vi "SpinAuxsAuto.vi"(6 "IntakeSpd":dbl, 7 "Time":dbl, 8 "error in":errorcluster, 9 "FeedSpd":dbl, 10 "Beltspd":dbl, 11 "ShootSpd":dbl) -> (0 "error out":errorcluster, 3 "Done":bool)   [LabVIEW 2020]
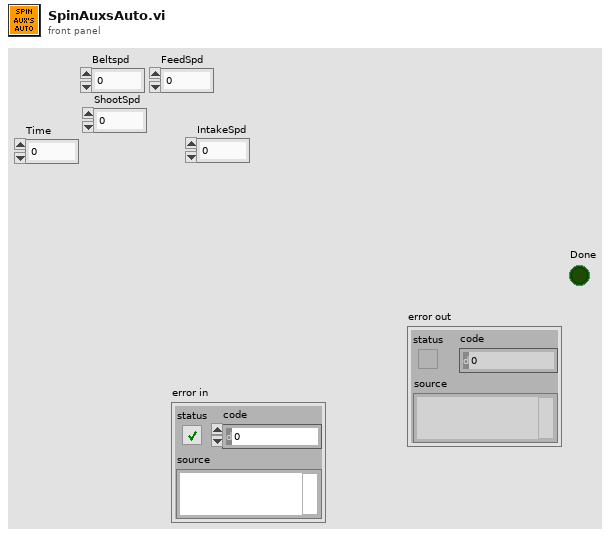
[diagram p1: front panel]
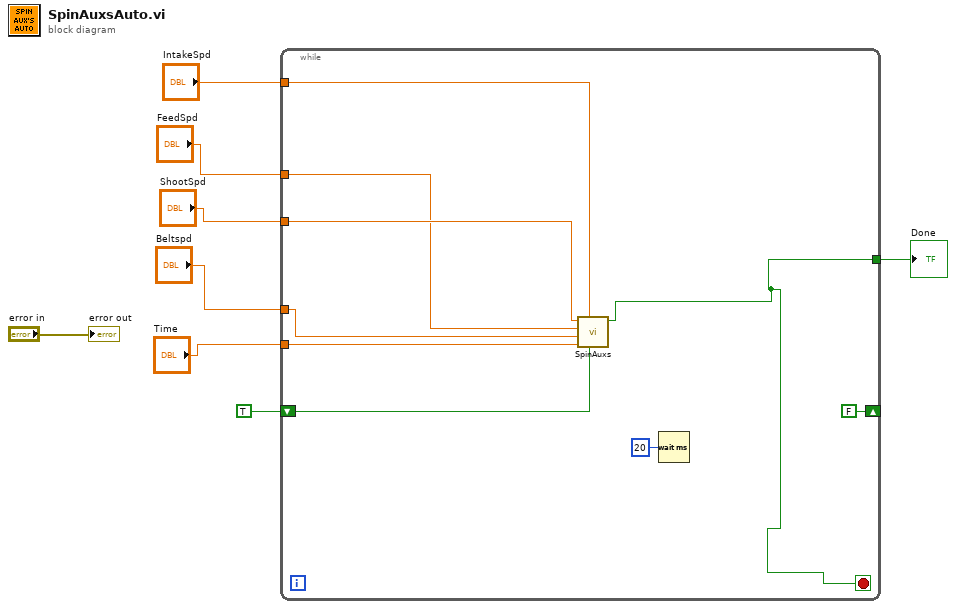
[diagram p0: block diagram]
diagram:
  n1 = while {
    tunnel: [w10] -> w7
    tunnel: "Beltspd" -> [w12]
    tunnel: "ShootSpd" -> [w14]
    tunnel: "FeedSpd" -> [w13]
    shift-right: [FALSE] -> _
    shift-left: TRUE -> [w11]
    tunnel: "Time" -> [w15]
    tunnel: "IntakeSpd" -> [w9]
    stop <- w10 stop-if-true
    n2 = call "SpinAuxs.vi"("Init"=w11, "IntakeSpeed"=w9, "Time"=w15, "BeltSpeed"=w12, "FeederSpeed"=w13, "ShootSpeed"=w14) -> ("Finished"=w10:bool)  [unwired: 4 in, 1 out]
    n3 = Wait (ms)(milliseconds to wait=u32 20) -> ()  [unwired: 1 out]
  }
  "Done" <- w7
  "error out" <- "error in"
